vi "ReadIniFiles_ByVarient.vi"(8 "error in (no error)":errorcluster, 10 "Varient":variant, 11 "path":path) -> (0 "error out":errorcluster, 3 "DataOut":variant)   [LabVIEW 2017]
uses:
  <vilib>/Utility/config.llb/NI_LVConfig.lvlib
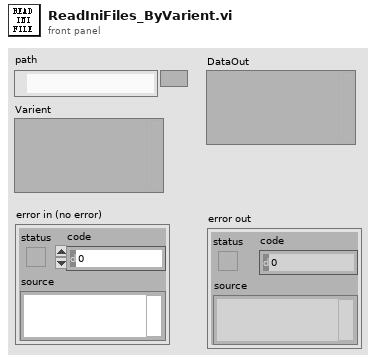
[diagram p1: front panel]
types:
  T1 = typedef "NI_LVConfig.lvlib/Config Data RefNum.ctl" = refnum<k1>
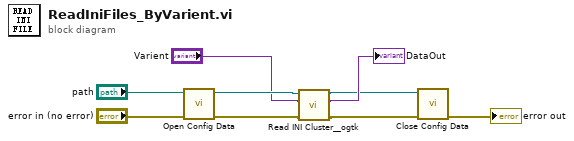
[diagram p0: block diagram]
diagram:
  n1 = call <vilib>:"Open Config Data.vi"("error in (no error)"="error in (no error)", "configuration file path"="path") -> ("error out"=w2:errorcluster, "refnum"=w6:T1)  [unwired: 7 in, 1 out]
  n2 = call "Read INI Cluster__ogtk.vi"("error in (no error)"=w2, "INI Fomatted Cluster Type"="Varient", "refnum"=w6) -> ("error out"=w1:errorcluster, "INI Fomatted Cluster"=→"DataOut":variant, "dup refnum"=w3:T1)  [unwired: 4 in, 2 out]
  n3 = call <vilib>:"Close Config Data.vi"("error in (no error)"=w1, "refnum"=w3) -> ("error out"=→"error out":errorcluster)  [unwired: 8 in, 1 out]
